vi "Init Complete Suite Message.vi"(5 "CompleteSuite Message":refnum<class "TestManagerMsg.CompleteSuite.lvclass">, 7 "overwrite?":bool=TRUE, 9 "notifier":refnum<notifier>, 10 "SuiteID":string, 11 "CallerID":string) -> (3 "Message":refnum<class "TestManagerMsg.lvclass">)   [LabVIEW 2020, in "Caraya.lvlib" / "TestManagerMsg.CompleteSuite.lvclass"]
uses:
  TestManagerMsg.CompleteSuite.lvclass
  C:/projects/caraya/src/classes/Test Manager Message/TestManagerMsg.lvclass
  Test Manager Message/TestManagerMsg.lvclass
  TestManagerMsg.CompleteSuite.lvclass/TestManagerMsg.CompleteSuite.ctl
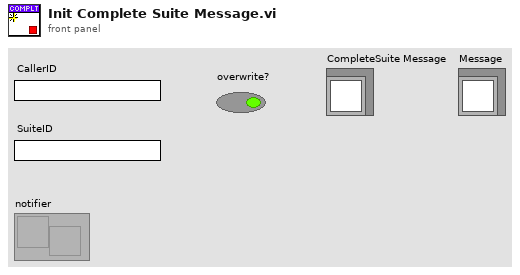
[diagram p1: front panel]
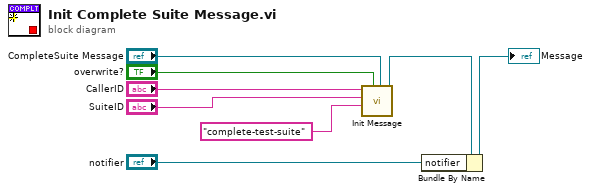
[diagram p0: block diagram]
diagram:
  n1 = call "Init Message.vi"("TestManagerMsg"="CompleteSuite Message", "overwrite?"="overwrite?", "key"="complete-test-suite" ("Message"), "self-id"="SuiteID", "owner-id"="CallerID") -> ("Message"=w7:refnum<class "TestManagerMsg.CompleteSuite.lvclass">)  [unwired: 6 in]
  n2 = Bundle By Name(cluster=w7, "notifier"="notifier") -> (→"Message":refnum<class "TestManagerMsg.CompleteSuite.lvclass">)
